vi "Load Status.vi"(8 "error in (no error)":errorcluster, 11 "Optics in":refnum<class "Optics.lvclass">) -> (0 "error out":errorcluster, 3 "Optics out":refnum<class "Optics.lvclass">)   [LabVIEW 2018, in "Optics.lvclass"]
uses:
  Optics.lvclass
  Optics.lvclass/Optics.ctl
panel:
  out "value":T1(array[cluster])
  in  "mechanisms in":T1(array[cluster])
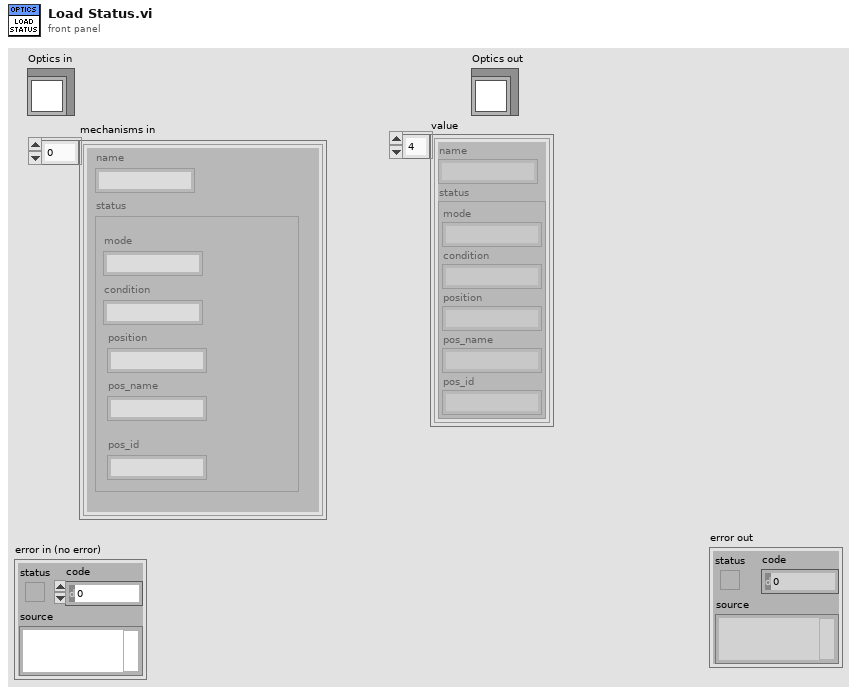
[diagram p1: front panel]
types:
  T1 = cluster{"name":string, "status":cluster{"mode":string, "condition":string, "position":string, "pos_name":string, "pos_id":string}}[]
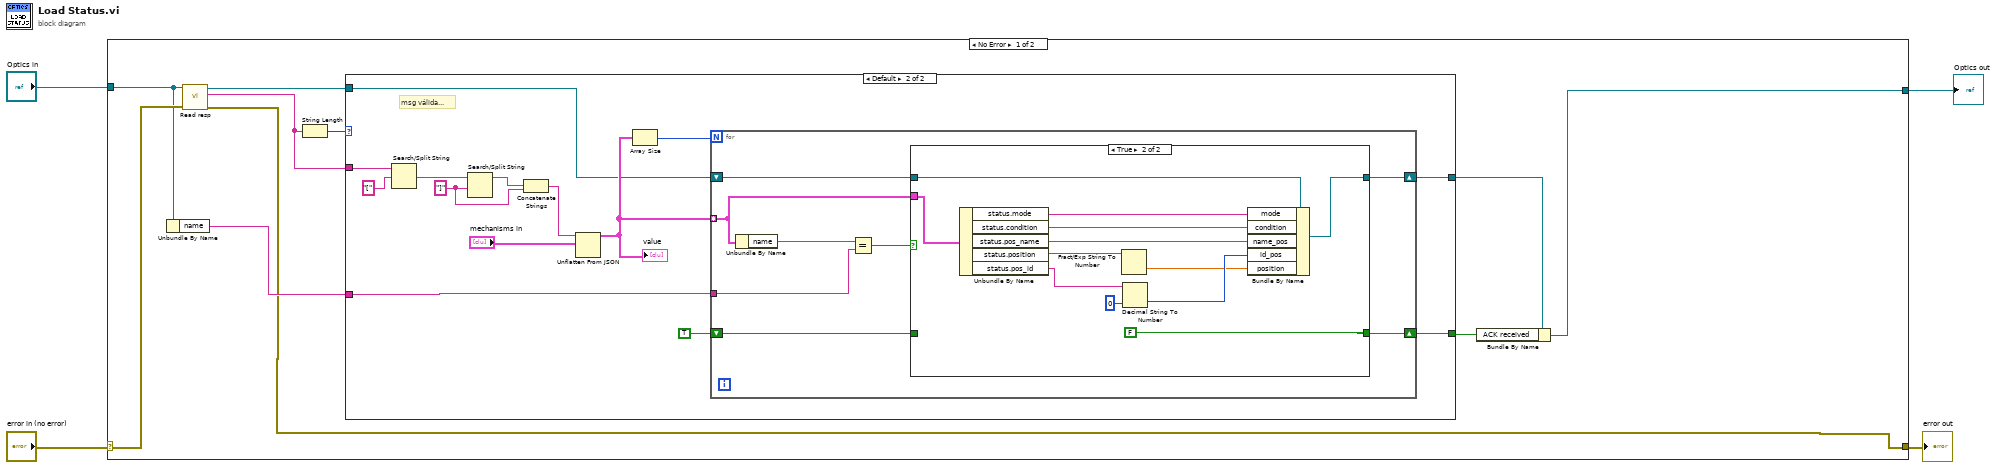
[diagram p0: block diagram]
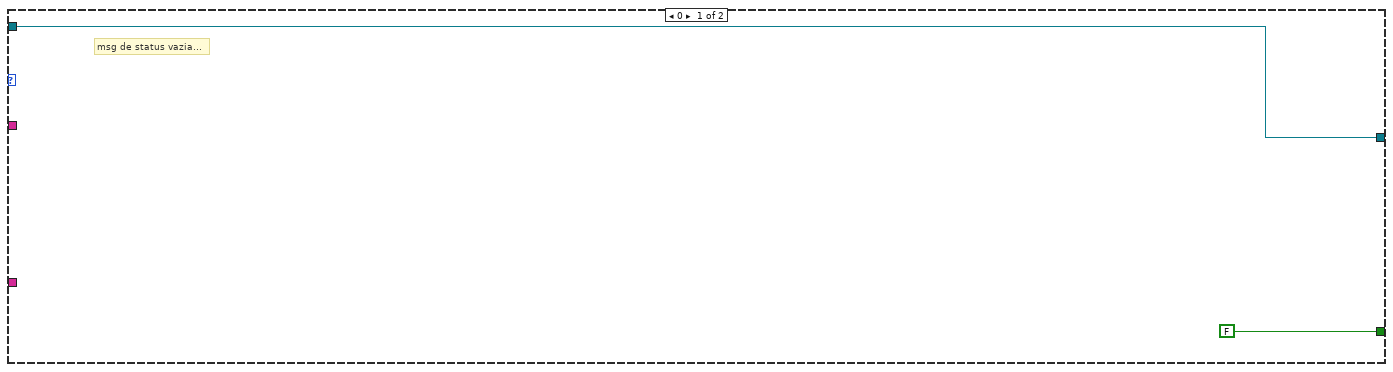
[diagram p2: hidden frame]
diagram:
  n1 = case shown="No Error" "error in (no error)" {
    selector: "error in (no error)" -> [w14 w54]
    tunnel: [w11 w54] -> w3
    tunnel: [w8 w53] -> w1
    tunnel: "Optics in" -> [w13 w53]
    frame No Error {
      n2 = Unbundle By Name(w13) -> ("name"=w12:string)
      n3 = call-dynamic "Read resp.vi"("error in (no error)"=w14, "Device in"=w13) -> ("error out"=w11:errorcluster, "resp"=w5:string, "Device out"=w10:refnum<class "Optics.lvclass">)  [unwired: 7 in]
      n4 = String Length(string=w5) -> (length=w6:i32)
      n5 = case shown="Default" w6 {
        tunnel: w5 -> [_ w30]
        tunnel: w12 -> [_ w29]
        tunnel: w10 -> [w16 w20]
        tunnel: [w16 w18] -> w9
        tunnel: [FALSE w17] -> w7
        frame 0 {
          # "msg de status vazia..."
        }
        frame Default {
          w26 = "]" ("search string/char (-)")
          # "msg válida..."
          n6 = Search/Split String(string=w30, search string/char (-)="[") -> (match + rest of string=w27:string)  [unwired: 1 in, 2 out]
          n7 = Search/Split String(string=w27, search string/char (-)=w26) -> (substring before match=w25:string)  [unwired: 1 in, 2 out]
          n8 = Concatenate Strings(w25, w26) -> (w24:string)
          n9 = Unflatten From JSON(JSON string=w24, type and defaults="mechanisms in") -> (value=w21:T1)  [unwired: 5 in, 1 out]
          "value" <- w21
          n10 = Array Size(array=w21) -> (size(s)=w22:i32)
          n11 = for {
            N: w22 -> [_]
            tunnel: w21 -> [w36] mode=indexing
            tunnel: w29 -> [w33]
            shift-right: [w31] -> w17
            shift-left: TRUE -> [w32]
            shift-right: [w34] -> w18
            shift-left: w20 -> [w35]
            n12 = Unbundle By Name(w36) -> ("name"=w38:string)
            n13 = Equal?(x=w38, y=w33) -> (x = y?=w37:bool)
            n14 = case shown="True" w37 {
              tunnel: w36 -> [_ w52]
              tunnel: w35 -> [w40 w43]
              tunnel: [w40 w41] -> w34
              tunnel: [w39 FALSE ("ACK received")] -> w31
              tunnel: w32 -> [w39 _]
              frame False {
              }
              frame True {
                n15 = Unbundle By Name(w52) -> ("status.mode"=w51:string, "status.condition"=w50:string, "status.pos_name"=w49:string, "status.position"=w48:string, "status.pos_id"=w47:string)
                n16 = Fract/Exp String To Number(string=w48) -> (number=w42:dbl)  [unwired: 3 in, 1 out]
                n17 = Decimal String To Number(string=w47, default (0L)=0 ("default (0 I32)")) -> (number=w46:i32)  [unwired: 1 in, 1 out]
                n18 = Bundle By Name(cluster=w43, "mode"=w51, "condition"=w50, "name_pos"=w49, "id_pos"=w46, "position"=w42) -> (w41:refnum<class "Optics.lvclass">)
              }
            }
          }
        }
      }
      n19 = Bundle By Name(cluster=w9, "ACK received"=w7) -> (w8:refnum<class "Optics.lvclass">)
    }
    frame Error {
    }
  }
  "error out" <- w3
  "Optics out" <- w1
